vi "FluxWrite.vi"(2 "Error In":errorcluster, 3 "Data":dbl, 4 "Função de Escrita":i32(ring) items=["Perform flowmeter zeroing", "Start/stop all totalizers", "Reset all totalizers", "Reset all inventories", "Mass flow rate meter factor", "Volume flow rate meter factor", "Density meter factor", "Flowing density calibration constant", "Mass flow scale factor", "Density scale factor", "Temperature scale factor", "Volume flow scale factor", "Pressure scale factor", "Mass total scale factor", "Volume total scale factor", "Mass inventory scale factor", "Volume inventory scale factor", "Standard or special mass flow unit", "Density unit", "Temperature unit", "Standard or special volume flow unit", "Pressure unit", "Standard or special mass total or inventory unit", "Standard or special volume total or inventory unit", "Base mass unit for special mass unit", "Base time uni for special mass unit", "Base volume unit for special volume unit", "Base time unit for special volume unit", "Maximum zeroing time", "Flow direction", "Perform transmitter self-test", "Mass flow cutoff", "Volume flow cutoff", "Slug flow high-density limit (g/cm3)", "Slug flow low-density limit (g/cm3)"], 5 "Master In":refnum<class "Modbus Master.lvclass">) -> (0 "Error Out":errorcluster, 1 "Master Out":refnum<class "Modbus Master.lvclass">)   [LabVIEW 2019]
uses:
  <vilib>/Modbus/master/Modbus Master.lvclass
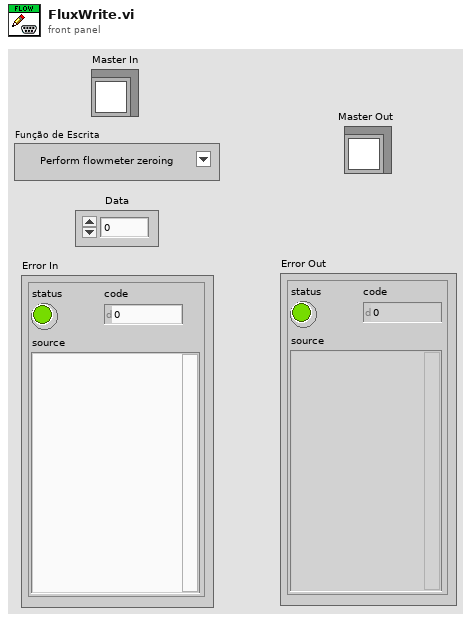
[diagram p1: front panel]
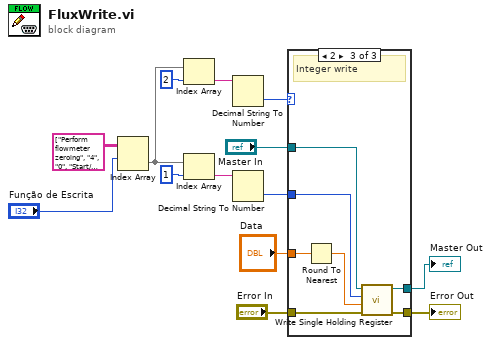
[diagram p0: block diagram]
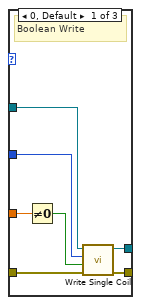
[diagram p2: hidden frame]
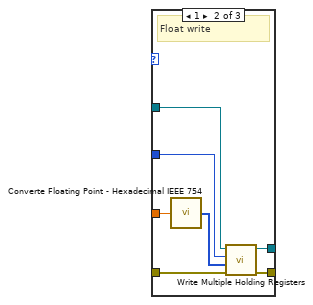
[diagram p3: hidden frame]
diagram:
  n1 = Index Array(array=string[][] [["Perform flowmeter zeroing", "4", "0"], ["Start/stop all totalizers", "1", "0"], ["Reset all totalizers", "2", "0"], ["Reset all inventories", "3", "0"], ["Mass flow rate meter factor", "278", "1"], ["Volume flow rate meter factor", "280", "1"], ["Density meter factor", "282", "1"], ["Flowing density calibration constant", "302", "1"], ["Mass flow scale factor", "28", "2"], ["Density scale factor", "29", "2"], ["Temperature scale factor", "30", "2"], ["Volume flow scale factor", "31", "2"], ["Pressure scale factor", "33", "2"], ["Mass total scale factor", "34", "2"], ["Volume total scale factor", "35", "2"], ["Mass inventory scale factor", "36", "2"], ["Volume inventory scale factor", "37", "2"], ["Standard or special mass flow unit", "38", "2"], ["Density unit", "39", "2"], ["Temperature unit", "40", "2"], ["Standard or special volume flow unit", "41", "2"], ["Pressure unit", "43", "2"], ["Standard or special mass total or inventory unit", "44", "2"], ["Standard or special volume total or inventory unit", "45", "2"], ["Base mass unit for special mass unit", "131", "2"], ["Base time uni for special mass unit", "132", "2"], ["Base volume unit for special volume unit", "133", "2"], ["Base time unit for special volume unit", "134", "2"], ["Maximum zeroing time", "135", "2"], ["Flow direction", "16", "2"], ["Perform transmitter self-test", "19", "0"], ["Mass flow cutoff", "194", "1"], ["Volume flow cutoff", "196", "1"], ["Slug flow high-density limit (g/cm3)", "198", "1"], ["Slug flow low-density limit (g/cm3)", "200", "1"]] ("Tabela de funções de escrita"), index (row)="Função de Escrita") -> (element=w9:string[])  [unwired: 1 in]
  n2 = Index Array(array=w9, index=2) -> (element=w10:string)
  n3 = Index Array(array=w9, index=1) -> (element=w11:string)
  n4 = Decimal String To Number(string=w10) -> (number=w4:i32)  [unwired: 2 in, 1 out]
  n5 = Decimal String To Number(string=w11) -> (number=w5:i32)  [unwired: 2 in, 1 out]
  n6 = case shown="2" w4 {
    tunnel: w5 -> [w21 w24 w31]
    tunnel: "Master In" -> [w20 w28 w35]
    tunnel: [w19 w27 w34] -> w1
    tunnel: [w18 w26 w33] -> w2
    tunnel: "Error In" -> [w17 w25 w32]
    tunnel: "Data" -> [w16 w22 w30]
    frame 0, Default {
      # "Boolean Write"
      n7 = Not Equal To 0?(x=w16) -> (x != 0?=w15:bool)
      n8 = call-dynamic "Write Single Coil.vi"("error in (no error)"=w17, "coil value"=w15, "address"=w21, "Modbus master in"=w20) -> ("error out"=w18:errorcluster, "Modbus master out"=w19:refnum<class "Modbus Master.lvclass">)  [unwired: 6 in]
    }
    frame 1 {
      # "Float write"
      n9 = call "Converte Floating Point - Hexadecimal IEEE 754.vi"("Floating point (entrada)"=w22) -> ("Array 2*[U16]"=w23:u16[])
      n10 = call-dynamic "Write Multiple Holding Registers.vi"("error in (no error)"=w25, "holding register values"=w23, "starting address"=w24, "Modbus master in"=w28) -> ("error out"=w26:errorcluster, "Modbus master out"=w27:refnum<class "Modbus Master.lvclass">)  [unwired: 6 in]
    }
    frame 2 {
      # "Integer write"
      n11 = Round To Nearest(number=w30) -> (nearest integer value=w29:dbl)
      n12 = call-dynamic "Write Single Holding Register.vi"("error in (no error)"=w32, "holding register value"=w29, "address"=w31, "Modbus master in"=w35) -> ("error out"=w33:errorcluster, "Modbus master out"=w34:refnum<class "Modbus Master.lvclass">)  [unwired: 6 in]
    }
  }
  "Master Out" <- w1
  "Error Out" <- w2
